vi "Write Data Output Setting.vi"(8 "error in (no error)":errorcluster, 10 "Data Output":enum16{"Resim", "Point Cloud"}(ring), 11 "LiDAR in":refnum<class "LiDAR.lvclass">) -> (0 "error out":errorcluster, 3 "LiDAR out":refnum<class "LiDAR.lvclass">)   [LabVIEW 2018]
uses:
  LiDAR.lvclass
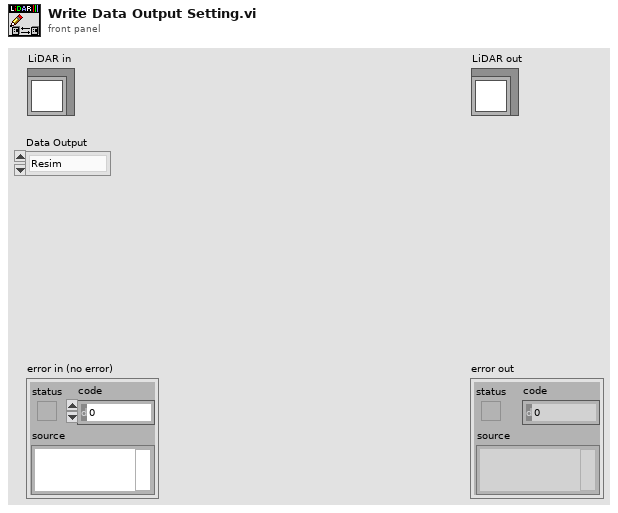
[diagram p1: front panel]
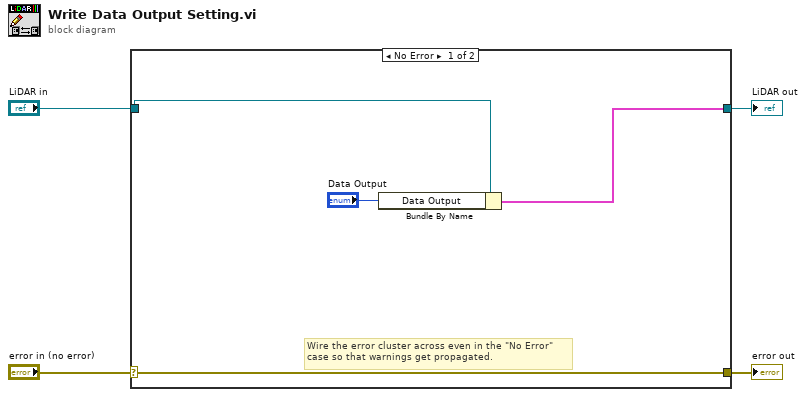
[diagram p0: block diagram]
diagram:
  n1 = case shown="No Error" "error in (no error)" {
    selector: "error in (no error)" -> [w8 w10]
    tunnel: [w8 w10] -> w3
    tunnel: [w6 w9] -> w1
    tunnel: "LiDAR in" -> [w7 w9]
    frame No Error {
      # "Wire the error cluster across even in the \"No Error\"\ncase so that warnings get propagated."
      n2 = Bundle By Name(cluster=w7, "Data Output"="Data Output") -> (w6:cluster{})
    }
    frame Error {
    }
  }
  "error out" <- w3
  "LiDAR out" <- w1
